vi "main.vi"() -> ()   [LabVIEW 2018]
uses:
  <vilib>/Math Plots/3D Math Plots/3D Contour/3D Contour XCtrl/3D Contour.xctl
  C:/Program Files (x86)/National Instruments/LabVIEW 2018/examples/Instrument IO/Serial/support/Serial - Settings.ctl
  <vilib>/Instr/_visa.llb/VISA Configure Serial Port (Instr).vi
  location_x.vi
  location_y.vi
  <instrlib>/Keithley 648X Series/Keithley 648X Series.lvlib
panel:
  out "Measurement":dbl
  in  "I-t开始":bool=TRUE
  in  "COM-WF Power":refnum<visa-resource-name>="COM4"
  out "说明":string="Y的最大移动范围为24 mm\nX最大移动范围23mm多一点"
  out "当前位置-Y":dbl
  out "当前位置-X":dbl
  in  "COM-Keithley":refnum<visa-resource-name>="GPIB0::22::INSTR"
  in  "程序停止":bool
  in  "COM-Y轴":refnum<visa-resource-name>="COM6"
  in  "Y回零":bool=TRUE
  in  "选项卡控件":T1(tab)
  in  "单动开始":bool=TRUE
  in  "Y轴单动":bool
  in  "移动距离(mm)":dbl=2.0 caption="元素" min=0.0 max=20.0 step=0.1
  in  "细分":u16=40000
  in  "速度(r/min)":u16=60
  in  "反向":bool=TRUE
  out "波形图表":dbl(graph)
  in  "线扫开始":bool=TRUE
  in  "Y轴线扫":bool
  out "XY图":cluster{"X":dbl, "Y":dbl}[](graph)
  in  "步长":dbl min=0.0 max=10.0 format="%#_13g"
  in  "距离":dbl min=0.0 max=20.0 format="%#_13g"
  in  "反向 2":bool=TRUE
  in  "二维扫描开始":bool=TRUE
  in  "Y起始":dbl format="%#_13g"
  in  "X步长":dbl format="%#_13g"
  in  "Y步长":dbl format="%#_13g"
  in  "X终止":dbl format="%#_13g"
  in  "Y终止":dbl format="%#_13g"
  in  "X起始":dbl format="%#_13g"
  in  "模块路径":path=path "D:/Github/Motor_ctrl/3d_plot.py"
  out "3D Contour":refnum<class "3D Plot Datatype.lvclass">[](xcontrol) caption="三维等高线"
  out "XY图 2":cluster{dbl[], dbl[]}(graph)
  in  "WF开始":bool=TRUE
  in  "Ramp Time (ms)":u32
  in  "Step V":dbl format="%#_13g"
  in  "End V":dbl format="%#_13g"
  in  "Start V":dbl format="%#_13g"
  in  "电压设置":bool=TRUE
  in  "V3 (+500)":sgl
  in  "V2 (-500)":sgl
  in  "V1 (-500)":sgl
  in  "V0 (+500)":sgl
  in  "DevIndex":i32
  in  "X回零":bool=TRUE
  in  "停止":bool=TRUE
  in  "COM-X轴":refnum<visa-resource-name>="COM5"
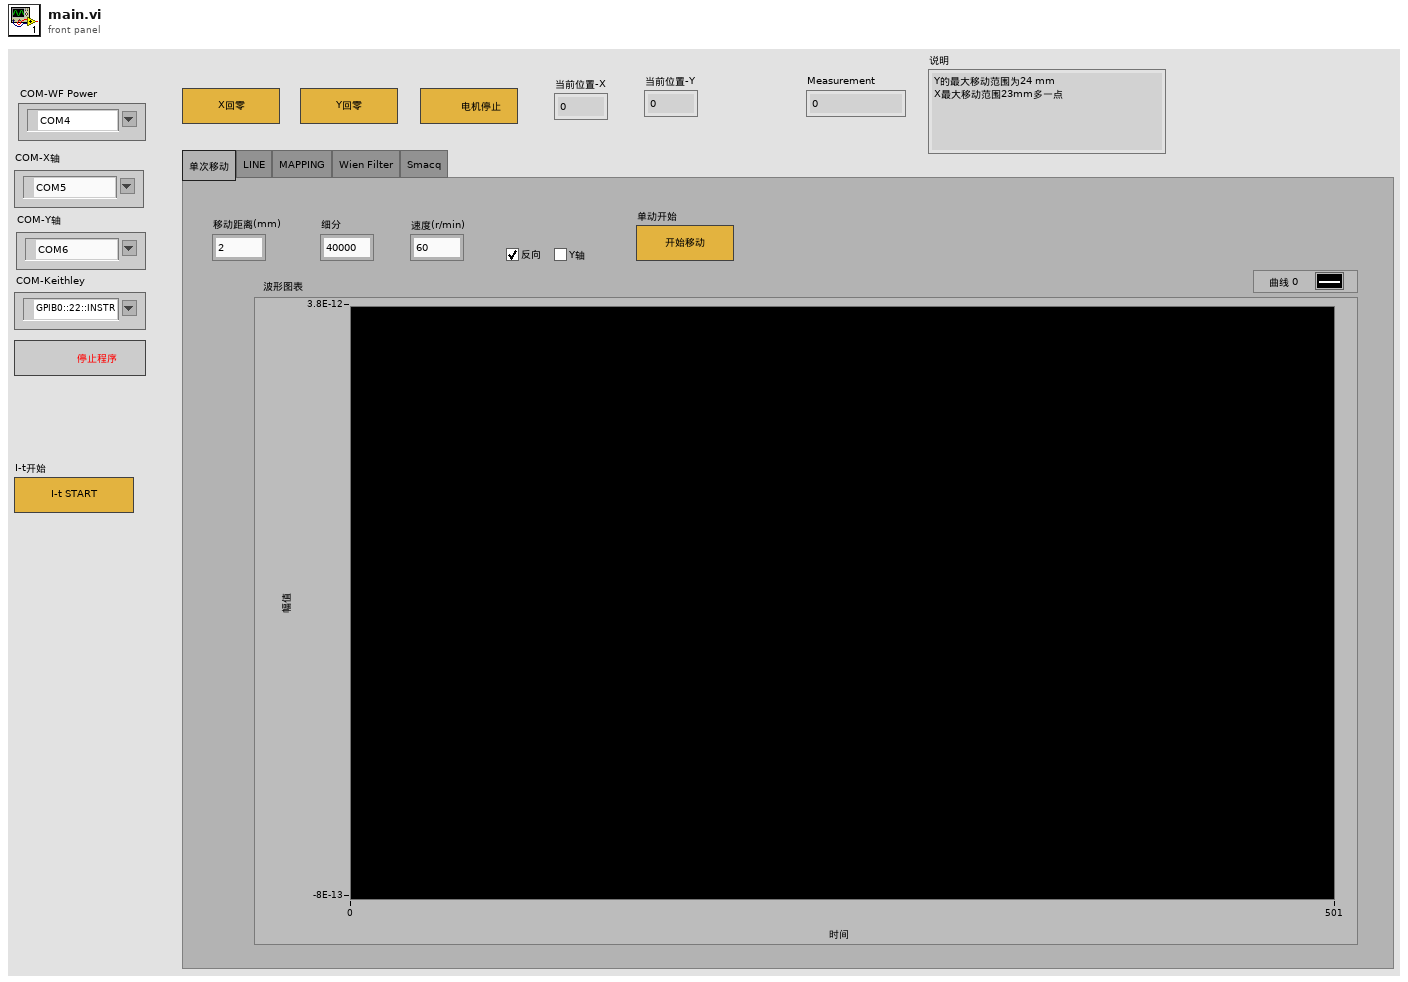
[diagram p1: front panel]
types:
  T1 = enum32{"单次移动", "LINE", "MAPPING", "Wien Filter", "Smacq"}
  T2 = cluster{"Baud Rate":u32, "Parity":u16, "Data Bits":u16, "Stop Bits":u16, "Flow Control":u16}
  T3 = typedef "Serial - Settings.ctl" = cluster{"波特率":u32, "数据位":u16, "校验":enum16{"None", "Odd", "Even", "Mark", "Space"}, "停止位":u16, "流控制":u16}
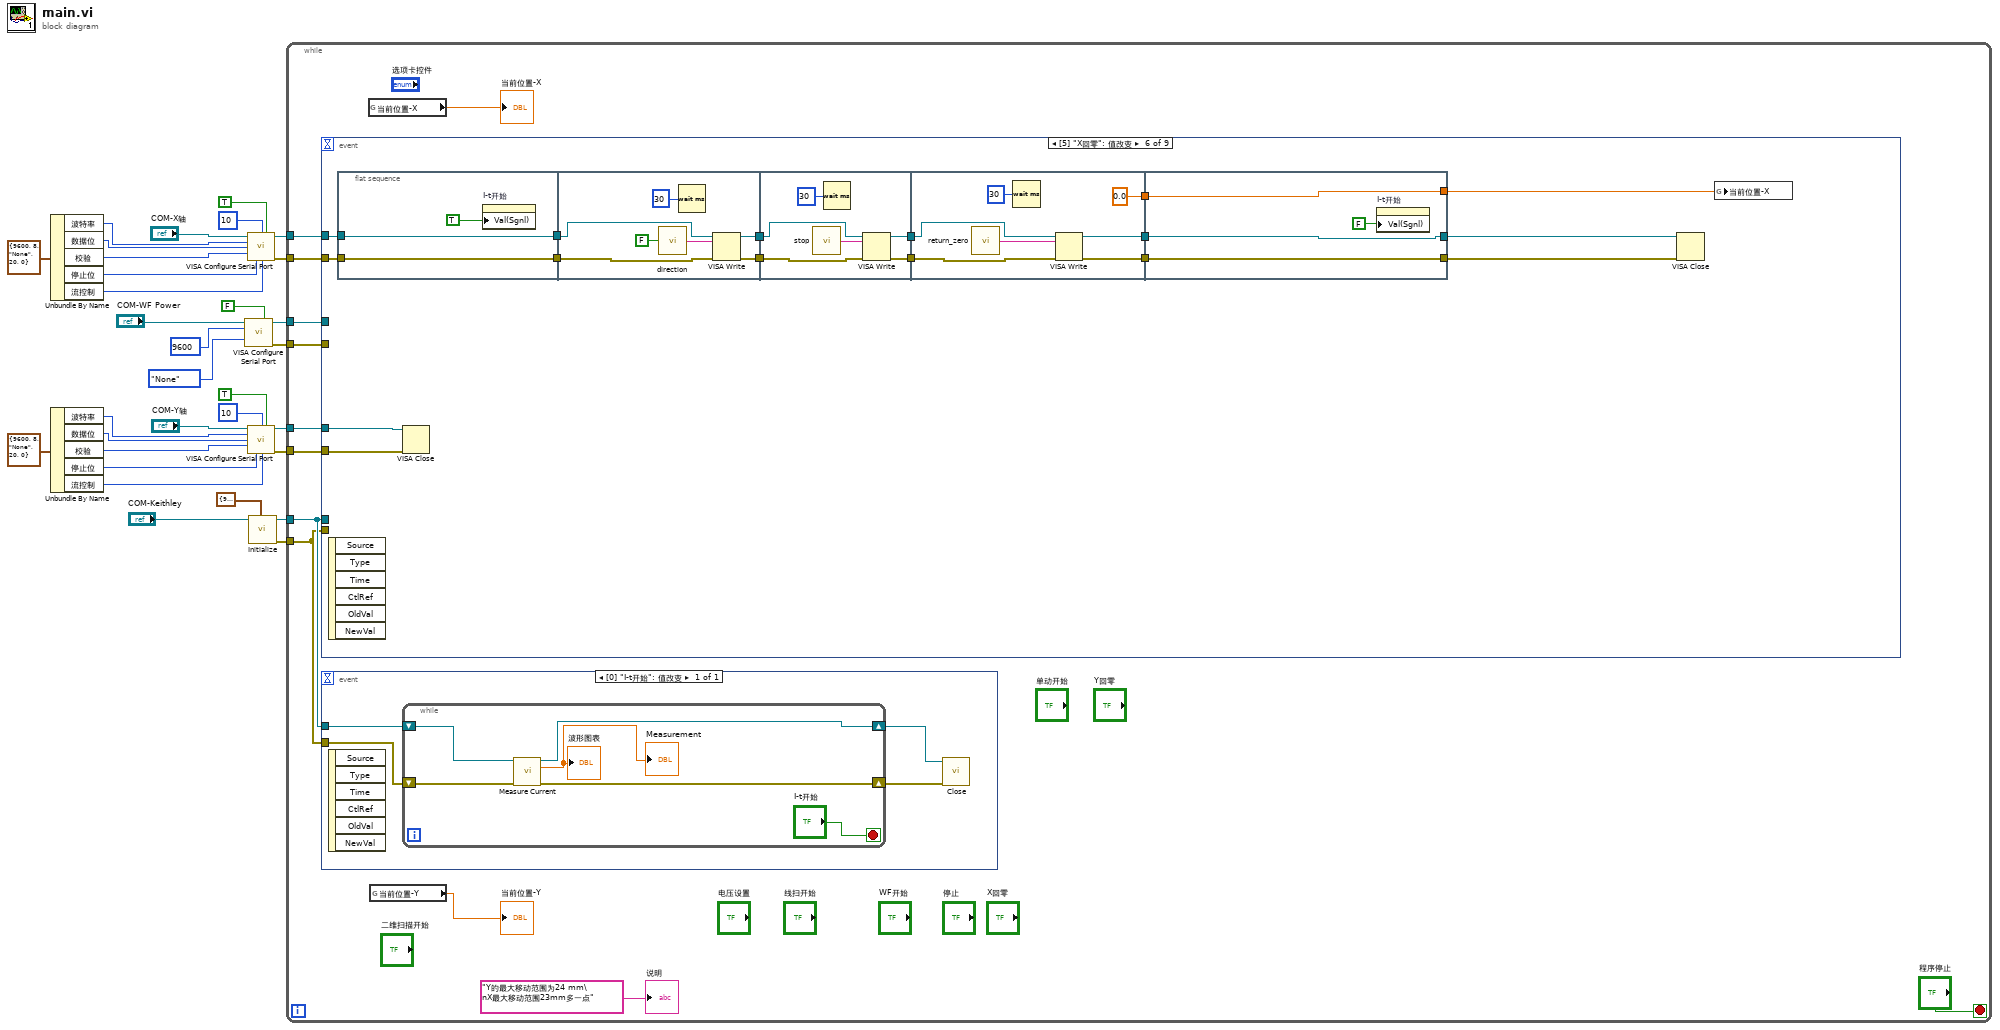
[diagram p0: block diagram]
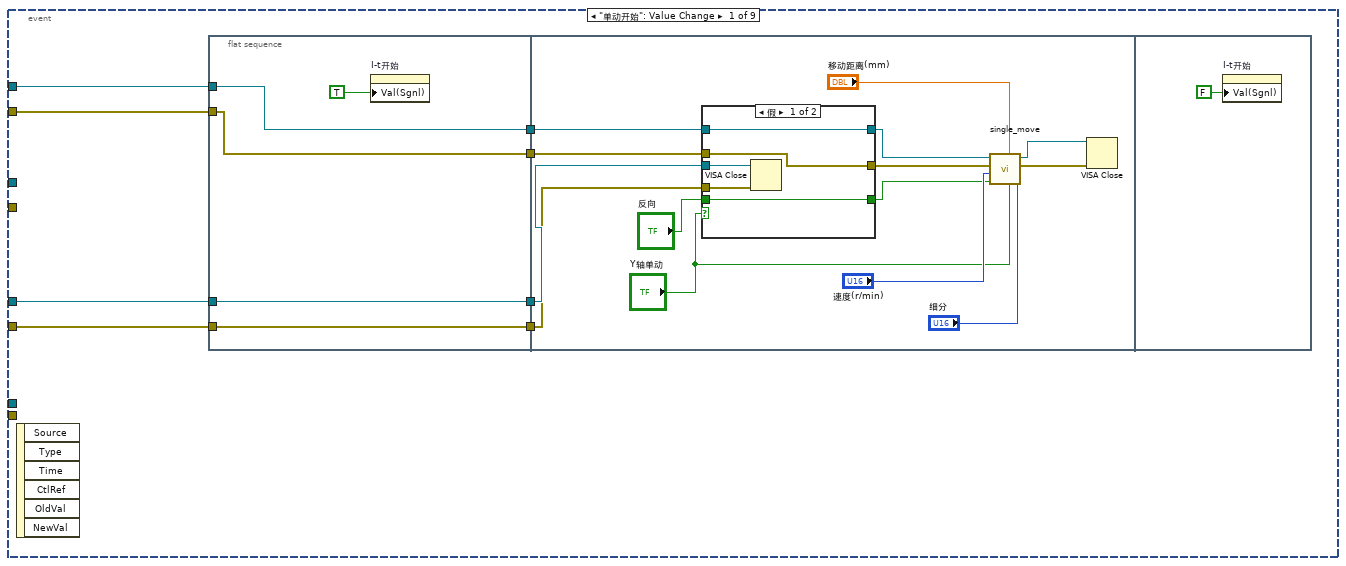
[diagram p2: hidden frame]
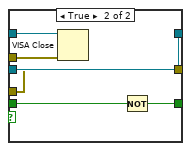
[diagram p3: hidden frame]
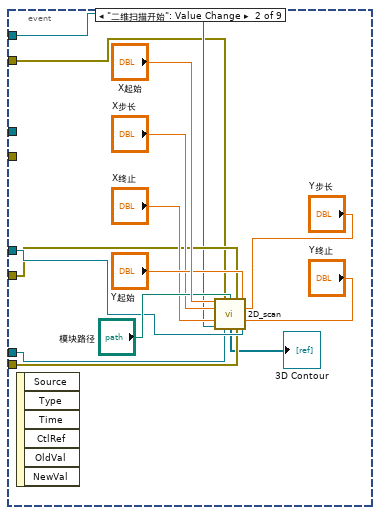
[diagram p4: hidden frame]
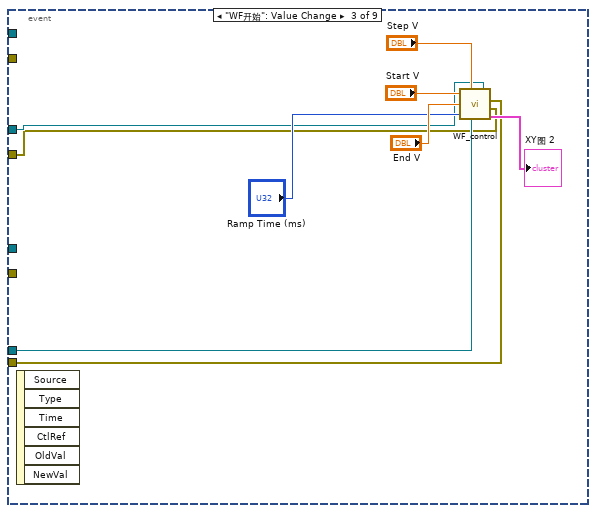
[diagram p5: hidden frame]
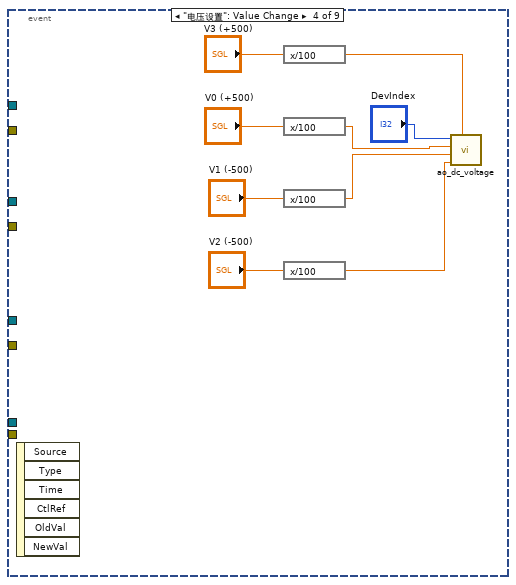
[diagram p6: hidden frame]
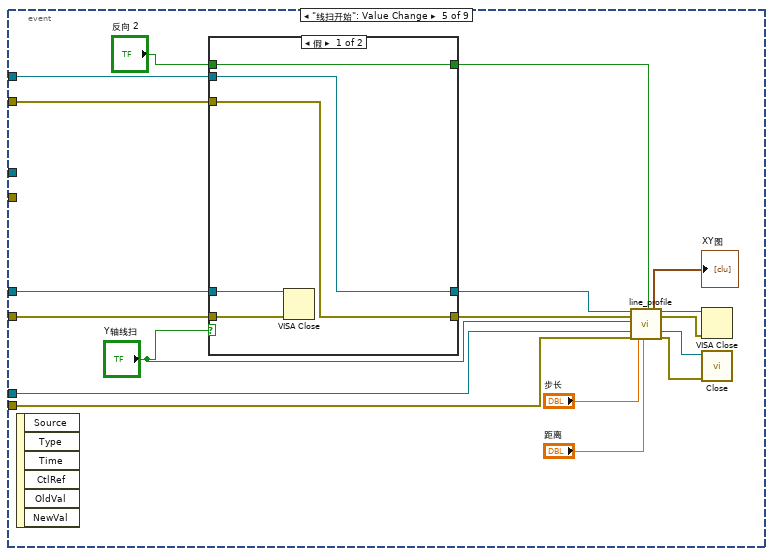
[diagram p7: hidden frame]
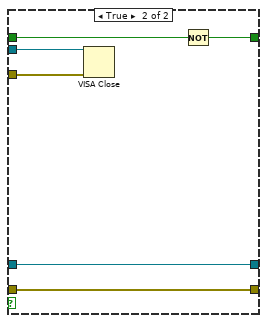
[diagram p8: hidden frame]
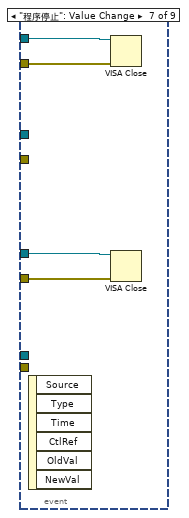
[diagram p9: hidden frame]
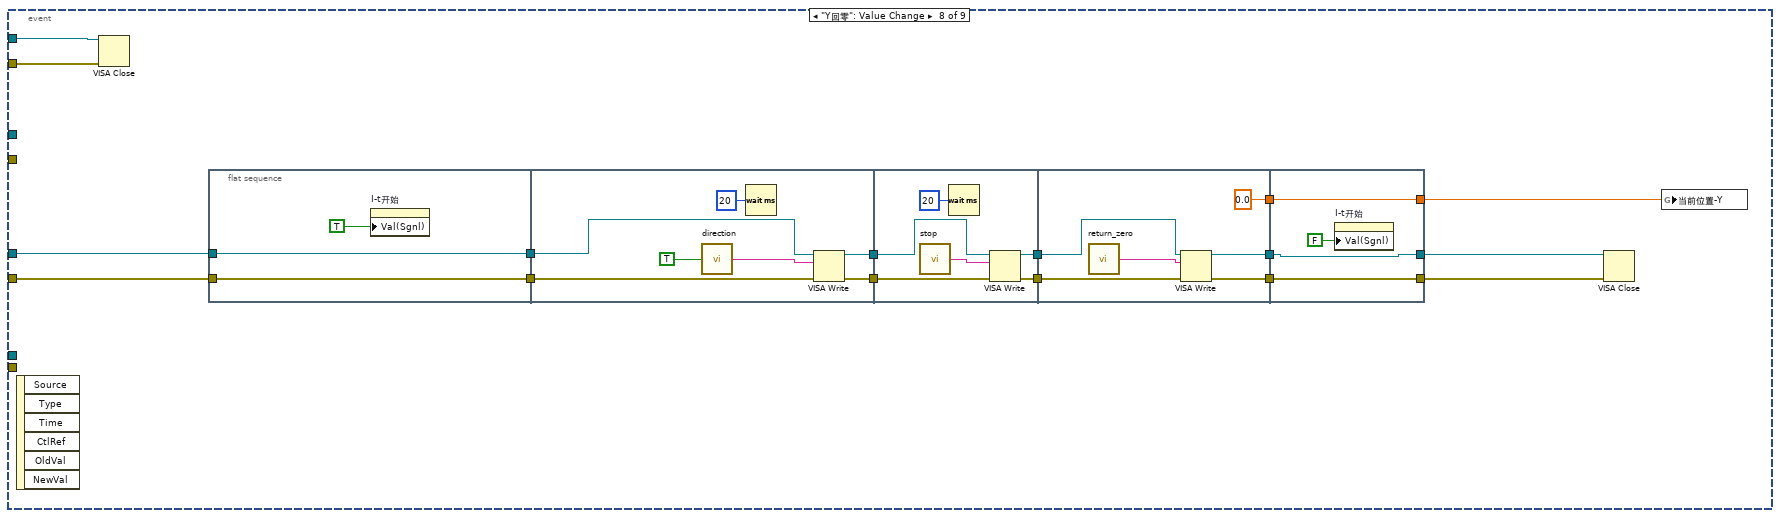
[diagram p10: hidden frame]
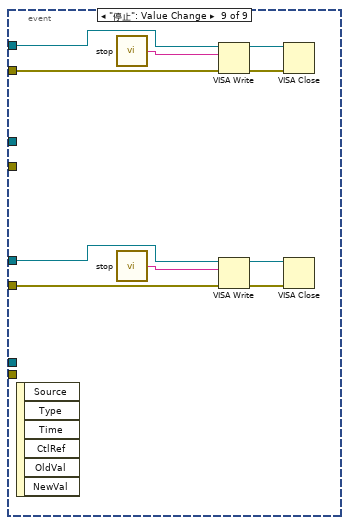
[diagram p11: hidden frame]
diagram:
  n1 = Unbundle By Name(T3 {"波特率"=9600, "数据位"=8, "校验"=enum."None", "停止位"=20, "流控制"=0} ("串口设置")) -> ("波特率"=w30:u32, "数据位"=w29:u16, "校验"=w28:enum16{"None", "Odd", "Even", "Mark", "Space"}, "停止位"=w27:u16, "流控制"=w26:u16)
  n2 = Unbundle By Name(T3 {"波特率"=9600, "数据位"=8, "校验"=enum."None", "停止位"=20, "流控制"=0} ("串口设置 2")) -> ("波特率"=w19:u32, "数据位"=w18:u16, "校验"=w17:enum16{"None", "Odd", "Even", "Mark", "Space"}, "停止位"=w16:u16, "流控制"=w15:u16)
  n3 = call-poly "VISA Configure Serial Port"("VISA resource name"="COM-WF Power", "Enable Termination\nChar (T)"=FALSE ("Enable Termination\nChar (T)"), "baud rate (9600)"=u32 9600, "parity (0:none)"=enum16{"None", "Odd", "Even", "Mark", "Space"}."None") -> ("VISA resource name out"=w2:refnum<visa-resource-name>, "error out"=w1:errorcluster)  [unwired: 10 in]
  n4 = call-poly "VISA Configure Serial Port"("VISA resource name"="COM-X轴", "termination char\n(0xA = '\\n' = LF)"=u8 10 ("termination char\n(0xA = '\\n' = LF)"), "Enable Termination\nChar (T)"=TRUE ("Enable Termination\nChar (T)"), "baud rate (9600)"=w30, "data bits (8)"=w29, "parity (0:none)"=w28, "stop bits (10: 1 bit)"=w27, "flow control (0:none)"=w26) -> ("VISA resource name out"=w22:refnum<visa-resource-name>, "error out"=w23:errorcluster)  [unwired: 2 in, 4 out]
  n5 = call-poly "VISA Configure Serial Port"("VISA resource name"="COM-Y轴", "termination char\n(0xA = '\\n' = LF)"=u8 10 ("termination char\n(0xA = '\\n' = LF)"), "Enable Termination\nChar (T)"=TRUE ("Enable Termination\nChar (T)"), "baud rate (9600)"=w19, "data bits (8)"=w18, "parity (0:none)"=w17, "stop bits (10: 1 bit)"=w16, "flow control (0:none)"=w15) -> ("VISA resource name out"=w12:refnum<visa-resource-name>, "error out"=w11:errorcluster)  [unwired: 2 in, 4 out]
  n6 = call <instrlib>:"Initialize.vi"("Serial Configuration"=T2 {"Baud Rate"=9600, "Parity"=0, "Data Bits"=8, "Stop Bits"=10, "Flow Control"=0}, "VISA resource name"="COM-Keithley") -> ("error out"=w8:errorcluster, "VISA resource name out"=w7:refnum<visa-resource-name>)  [unwired: 8 in]
  n7 = while {
    tunnel: w23 -> [w44]
    tunnel: w22 -> [w43]
    tunnel: w12 -> [w42]
    tunnel: w11 -> [w41]
    tunnel: w8 -> [w37]
    tunnel: w7 -> [w38]
    tunnel: w2 -> [w40]
    tunnel: w1 -> [w39]
    stop <- "程序停止" stop-if-true
    n8 = event shown="[5] \"X回零\": 值改变" {
      selector: _ -> [_ _ _ _ _ _ _ _ _]
      dyn-events: _ -> [_ _ _ _ _ _ _ _ _]
      timeout: _ -> [_ _ _ _ _ _ _ _ _]
      tunnel: w44 -> [w59 w97 _ _ w142 w169 w198 w210 w251]
      tunnel: w43 -> [w60 w98 _ _ w143 w170 w199 w211 w252]
      tunnel: w42 -> [w62 w100 _ _ w141 w164 w201 w215 w249]
      tunnel: w41 -> [w61 w99 _ _ w140 w163 w200 w214 w248]
      tunnel: w37 -> [_ w95 w111 _ w136 _ _ _ _]
      tunnel: w38 -> [_ w96 w110 _ w137 _ _ _ _]
      tunnel: w40 -> [_ _ w109 _ _ _ _ _ _]
      tunnel: w39 -> [_ _ w108 _ _ _ _ _ _]
      event "单动开始": Value Change {
        n9 = event-data() -> ()  [unwired: 1 in, 6 out]
        n10 = flat-sequence {
          tunnel: w59 -> [w64]
          tunnel: w60 -> [w65]
          tunnel: w61 -> [w66]
          tunnel: w62 -> [w67]
          tunnel: [w67] -> w58
          tunnel: [w66] -> w57
          tunnel: [w65] -> w56
          tunnel: [w64] -> w55
          tunnel: w58 -> [w81]
          tunnel: w57 -> [w80]
          tunnel: w56 -> [w79]
          tunnel: w55 -> [w78]
          frame #0 {
            n11 = property on="I-t开始" class="Bool (严格)"("Val(Sgnl)"=TRUE ("值(信号)")) -> ()  [unwired: 2 in, 2 out]
          }
          frame #1 {
            n12 = case shown="假" "Y轴单动" {
              tunnel: [w86 w92] -> w77
              tunnel: w81 -> [w84 w92]
              tunnel: [w85 w91] -> w76
              tunnel: w80 -> [w83 w91]
              tunnel: w79 -> [w86 w90]
              tunnel: w78 -> [w85 w89]
              tunnel: "反向" -> [w82 w88]
              tunnel: [w82 w87] -> w68
              frame False {
                n13 = VISA Close(VISA resource name=w84, error in (no error)=w83) -> ()  [unwired: 1 out]
              }
              frame True {
                n14 = VISA Close(VISA resource name=w90, error in (no error)=w89) -> ()  [unwired: 1 out]
                n15 = Not(x=w88) -> (.not. x?=w87:bool)
              }
            }
            n16 = call "single_move.vi"("COM In"=w77, "error In"=w76, "速度(r/min)"="速度(r/min)", "反向"=w68, "移动距离(mm)"="移动距离(mm)", "Y轴"="Y轴单动", "细分"="细分") -> ("VISA resource name out 2"=w75:refnum<visa-resource-name>, "error out 2"=w74:errorcluster)  [unwired: 1 out]
            n17 = VISA Close(VISA resource name=w75, error in (no error)=w74) -> ()  [unwired: 1 out]
          }
          frame #2 {
            n18 = property on="I-t开始" class="Bool (严格)"("Val(Sgnl)"=FALSE) -> ()  [unwired: 2 in, 2 out]
          }
        }
      }
      event "二维扫描开始": Value Change {
        n19 = event-data() -> ()  [unwired: 1 in, 6 out]
        n20 = call "2D_scan.vi"("X起始"="X起始", "ERR X"=w97, "模块路径"="模块路径", "ERR Y"=w99, "Y起始"="Y起始", "X步长"="X步长", "Y步长"="Y步长", "X终止"="X终止", "Y终止"="Y终止", "COM X"=w98, "COM Keithley"=w96, "ERR Keithley"=w95, "COM Y"=w100) -> ("3D Plot lvclass Array out"=→"3D Contour":refnum<class "3D Plot Datatype.lvclass">[])  [unwired: 2 in]
      }
      event "WF开始": Value Change {
        n21 = event-data() -> ()  [unwired: 1 in, 6 out]
        n22 = call "WF_control.vi"("Start V"="Start V", "Step V"="Step V", "End V"="End V", "Ramp Time (ms)"="Ramp Time (ms)", "COM Keithley"=w110, "COM WF"=w109, "ERR Keithley"=w111, "ERR WF"=w108) -> ("XY图"=→"XY图 2":cluster{dbl[], dbl[]})
      }
      event "电压设置": Value Change {
        n23 = event-data() -> ()  [unwired: 1 in, 6 out]
        n24 = expression code="x/100"("V3 (+500)") -> (w120:sgl)
        n25 = expression code="x/100"("V0 (+500)") -> (w119:sgl)
        n26 = expression code="x/100"("V1 (-500)") -> (w118:sgl)
        n27 = expression code="x/100"("V2 (-500)") -> (w117:sgl)
        n28 = call <instrlib>:"ao_dc_voltage.vi"("Voltage 3"=w120, "Voltage 2"=w117, "Voltage 1"=w118, "Voltage 0"=w119, "DevIndex"="DevIndex") -> ()  [unwired: 7 in]
      }
      event "线扫开始": Value Change {
        n29 = event-data() -> ()  [unwired: 1 in, 6 out]
        n30 = case shown="假" "Y轴线扫" {
          tunnel: [w148 w154] -> w139
          tunnel: w143 -> [w148 w152]
          tunnel: [w147 w153] -> w138
          tunnel: w142 -> [w147 w151]
          tunnel: w141 -> [w146 w154]
          tunnel: w140 -> [w145 w153]
          tunnel: "反向 2" -> [w144 w150]
          tunnel: [w144 w149] -> w126
          frame False {
            n31 = VISA Close(VISA resource name=w146, error in (no error)=w145) -> ()  [unwired: 1 out]
          }
          frame True {
            n32 = VISA Close(VISA resource name=w152, error in (no error)=w151) -> ()  [unwired: 1 out]
            n33 = Not(x=w150) -> (.not. x?=w149:bool)
          }
        }
        n34 = call "line_profile.vi"("Motor COM in"=w139, "Motor error in"=w138, "Y轴"="Y轴线扫", "Keithley COM In"=w137, "Keithley Error In"=w136, "步长"="步长", "距离"="距离", "反向"=w126) -> ("XY图"=→"XY图":cluster{"X":dbl, "Y":dbl}[], "Motor COM out"=w132:refnum<visa-resource-name>, "Motor error out"=w131:errorcluster, "Keithley COM out"=w130:refnum<visa-resource-name>, "Keithley Error out"=w129:errorcluster)  [unwired: 4 in, 3 out]
        n35 = VISA Close(VISA resource name=w132, error in (no error)=w131) -> ()  [unwired: 1 out]
        n36 = call <instrlib>:"Close.vi"("error in (no error)"=w129, "VISA resource name"=w130) -> ()  [unwired: 9 in, 1 out]
      }
      event "X回零": Value Change {
        n37 = event-data() -> ()  [unwired: 1 in, 6 out]
        n38 = flat-sequence {
          tunnel: w169 -> [w172]
          tunnel: w170 -> [w173]
          tunnel: [w173] -> w159
          tunnel: [w172] -> w158
          tunnel: [w179] -> w162
          tunnel: [w177] -> w161
          tunnel: w159 -> [w180]
          tunnel: w158 -> [w178]
          tunnel: [w185] -> w168
          tunnel: [w183] -> w167
          tunnel: w162 -> [w186]
          tunnel: w161 -> [w184]
          tunnel: w168 -> [w193]
          tunnel: w167 -> [w192]
          tunnel: [0.0] -> w157
          tunnel: [w188] -> w156
          tunnel: [w187] -> w155
          tunnel: [w197] -> w160
          tunnel: [w195] -> w166
          tunnel: [w194] -> w165
          tunnel: w157 -> [w197]
          tunnel: w156 -> [w195]
          tunnel: w155 -> [w194]
          frame #0 {
            n39 = property on="I-t开始" class="Bool (严格)"("Val(Sgnl)"=TRUE ("值(信号)")) -> ()  [unwired: 2 in, 2 out]
          }
          frame #1 {
            n40 = call "direction.vi"("反向"=FALSE) -> ("指令"=w176:string)
            n41 = Wait (ms)(milliseconds to wait=u32 30 ("等待时间（毫秒）")) -> ()  [unwired: 1 out]
            n42 = VISA Write(VISA resource name=w180, write buffer=w176, error in (no error)=w178) -> (VISA resource name out=w179:refnum<visa-resource-name>, error out=w177:errorcluster)  [unwired: 1 out]
          }
          frame #2 {
            n43 = call "stop.vi"() -> ("指令"=w182:string)
            n44 = Wait (ms)(milliseconds to wait=u32 30 ("等待时间（毫秒）")) -> ()  [unwired: 1 out]
            n45 = VISA Write(VISA resource name=w186, write buffer=w182, error in (no error)=w184) -> (VISA resource name out=w185:refnum<visa-resource-name>, error out=w183:errorcluster)  [unwired: 1 out]
          }
          frame #3 {
            n46 = call "return_zero.vi"() -> ("指令"=w191:string)
            n47 = Wait (ms)(milliseconds to wait=u32 30 ("等待时间（毫秒）")) -> ()  [unwired: 1 out]
            n48 = VISA Write(VISA resource name=w193, write buffer=w191, error in (no error)=w192) -> (VISA resource name out=w188:refnum<visa-resource-name>, error out=w187:errorcluster)  [unwired: 1 out]
          }
          frame #4 {
            n49 = property on="I-t开始" class="Bool (严格)"("Val(Sgnl)"=FALSE ("值(信号)")) -> ()  [unwired: 2 in, 2 out]
          }
        }
        n50 = VISA Close(VISA resource name=w164, error in (no error)=w163) -> ()  [unwired: 1 out]
        n51 = VISA Close(VISA resource name=w166, error in (no error)=w165) -> ()  [unwired: 1 out]
        n52 = global write "location_x.vi" "当前位置-X"(w160) -> ()
      }
      event "程序停止": Value Change {
        n53 = event-data() -> ()  [unwired: 1 in, 6 out]
        n54 = VISA Close(VISA resource name=w199, error in (no error)=w198) -> ()  [unwired: 1 out]
        n55 = VISA Close(VISA resource name=w201, error in (no error)=w200) -> ()  [unwired: 1 out]
      }
      event "Y回零": Value Change {
        n56 = event-data() -> ()  [unwired: 1 in, 6 out]
        n57 = VISA Close(VISA resource name=w211, error in (no error)=w210) -> ()  [unwired: 1 out]
        n58 = flat-sequence {
          tunnel: w214 -> [w219]
          tunnel: w215 -> [w220]
          tunnel: [w220] -> w206
          tunnel: [w219] -> w205
          tunnel: [w224] -> w209
          tunnel: [w222] -> w208
          tunnel: w206 -> [w225]
          tunnel: w205 -> [w223]
          tunnel: [w232] -> w217
          tunnel: [w230] -> w216
          tunnel: w209 -> [w233]
          tunnel: w208 -> [w231]
          tunnel: w217 -> [w239]
          tunnel: w216 -> [w238]
          tunnel: [w237] -> w204
          tunnel: [w236] -> w203
          tunnel: [0.0] -> w202
          tunnel: [w241] -> w207
          tunnel: [w242] -> w213
          tunnel: [w243] -> w212
          tunnel: w204 -> [w243]
          tunnel: w203 -> [w242]
          tunnel: w202 -> [w241]
          frame #0 {
            n59 = property on="I-t开始" class="Bool (严格)"("Val(Sgnl)"=TRUE ("值(信号)")) -> ()  [unwired: 2 in, 2 out]
          }
          frame #1 {
            n60 = call "direction.vi"("反向"=TRUE) -> ("指令"=w227:string)
            n61 = Wait (ms)(milliseconds to wait=u32 20 ("等待时间（毫秒）")) -> ()  [unwired: 1 out]
            n62 = VISA Write(VISA resource name=w225, write buffer=w227, error in (no error)=w223) -> (VISA resource name out=w224:refnum<visa-resource-name>, error out=w222:errorcluster)  [unwired: 1 out]
          }
          frame #2 {
            n63 = call "stop.vi"() -> ("指令"=w229:string)
            n64 = Wait (ms)(milliseconds to wait=u32 20 ("等待时间（毫秒）")) -> ()  [unwired: 1 out]
            n65 = VISA Write(VISA resource name=w233, write buffer=w229, error in (no error)=w231) -> (VISA resource name out=w232:refnum<visa-resource-name>, error out=w230:errorcluster)  [unwired: 1 out]
          }
          frame #3 {
            n66 = call "return_zero.vi"() -> ("指令"=w235:string)
            n67 = VISA Write(VISA resource name=w239, write buffer=w235, error in (no error)=w238) -> (VISA resource name out=w236:refnum<visa-resource-name>, error out=w237:errorcluster)  [unwired: 1 out]
          }
          frame #4 {
            n68 = property on="I-t开始" class="Bool (严格)"("Val(Sgnl)"=FALSE ("值(信号)")) -> ()  [unwired: 2 in, 2 out]
          }
        }
        n69 = VISA Close(VISA resource name=w213, error in (no error)=w212) -> ()  [unwired: 1 out]
        n70 = global write "location_y.vi" "当前位置-Y"(w207) -> ()
      }
      event "停止": Value Change {
        n71 = event-data() -> ()  [unwired: 1 in, 6 out]
        n72 = call "stop.vi"() -> ("指令"=w253:string)
        n73 = call "stop.vi"() -> ("指令"=w250:string)
        n74 = VISA Write(VISA resource name=w252, write buffer=w253, error in (no error)=w251) -> (VISA resource name out=w246:refnum<visa-resource-name>, error out=w245:errorcluster)  [unwired: 1 out]
        n75 = VISA Write(VISA resource name=w249, write buffer=w250, error in (no error)=w248) -> (VISA resource name out=w247:refnum<visa-resource-name>, error out=w244:errorcluster)  [unwired: 1 out]
        n76 = VISA Close(VISA resource name=w246, error in (no error)=w245) -> ()  [unwired: 1 out]
        n77 = VISA Close(VISA resource name=w247, error in (no error)=w244) -> ()  [unwired: 1 out]
      }
    }
    n78 = event shown="[0] \"I-t开始\": 值改变" {
      selector: _ -> [_]
      dyn-events: _ -> [_]
      timeout: _ -> [_]
      tunnel: w38 -> [w48]
      tunnel: w37 -> [w47]
      event "I-t开始": Value Change {
        n79 = event-data() -> ()  [unwired: 1 in, 6 out]
        n80 = while {
          shift-right: [w49] -> w45
          shift-left: w48 -> [w54]
          shift-right: [w52] -> w46
          shift-left: w47 -> [w53]
          stop <- "I-t开始" stop-if-true
          n81 = call <instrlib>:"Measure Current.vi"("VISA resource name"=w54, "error in (no error)"=w53) -> ("VISA resource name out"=w49:refnum<visa-resource-name>, "Measurement"=→"Measurement" →"波形图表":dbl, "error out"=w52:errorcluster)  [unwired: 11 in]
        }
        n82 = call <instrlib>:"Close.vi"("error in (no error)"=w46, "VISA resource name"=w45) -> ()  [unwired: 9 in, 1 out]
      }
    }
    n83 = global read "location_x.vi" "当前位置-X"() -> (→"当前位置-X":dbl)
    n84 = global read "location_y.vi" "当前位置-Y"() -> (→"当前位置-Y":dbl)
    "说明" <- "Y的最大移动范围为24 mm\nX最大移动范围23mm多一点" ("字符串")
  }
